vi "WriteMultimeterDarkVoltage.vi"(8 "error in (no error)":errorcluster, 10 "Dark Voltage":dbl, 11 "MultimeterSim in":refnum<class "MultimeterSim.lvclass">) -> (0 "error out":errorcluster, 3 "MultimeterSim out":refnum<class "MultimeterSim.lvclass">)   [LabVIEW 2017, in "MultimeterSim.lvclass"]
uses:
  MultimeterSim.lvclass
  MultimeterSim.lvclass/MultimeterSim.ctl
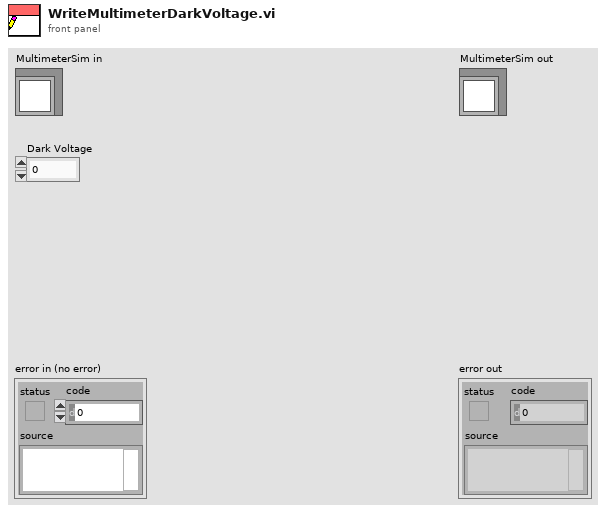
[diagram p1: front panel]
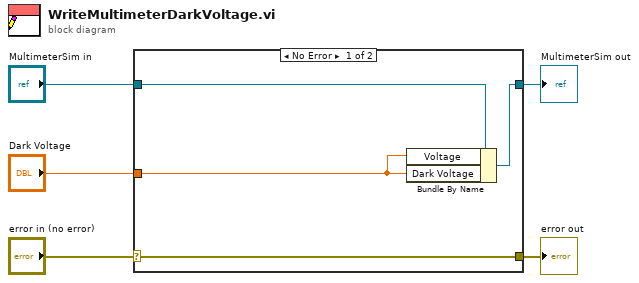
[diagram p0: block diagram]
diagram:
  n1 = case shown="No Error" "error in (no error)" {
    selector: "error in (no error)" -> [w9 w10]
    tunnel: [w9 w10] -> w4
    tunnel: [w7 w11] -> w2
    tunnel: "MultimeterSim in" -> [w8 w11]
    tunnel: "Dark Voltage" -> [w6 _]
    frame No Error {
      n2 = Bundle By Name(cluster=w8, "Voltage"=w6, "Dark Voltage"=w6) -> (w7:refnum<class "MultimeterSim.lvclass">)
    }
    frame Error {
    }
  }
  "error out" <- w4
  "MultimeterSim out" <- w2
